vi "Load Dark Array Data.vi"(8 "error in (no error)":errorcluster, 11 "Dark Array Path":path) -> (0 "error out":errorcluster, 1 "Freq":dbl[](array[numeric]), 2 "intTime":dbl[](array[numeric]), 3 "Scans":dbl[][](array[numeric]))   [LabVIEW 2014, in "AvaSpec.lvlib" / "Dark.lvlib"]
uses:
  Dark.lvlib
  AvaSpec.lvlib
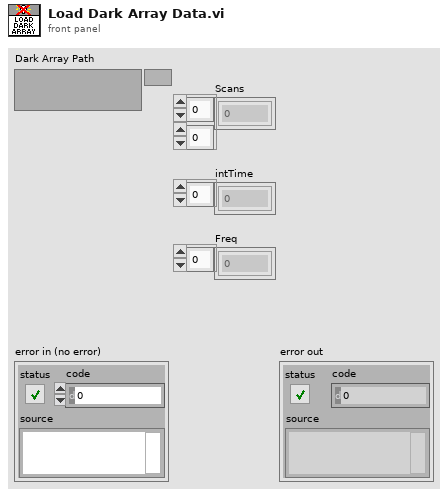
[diagram p1: front panel]
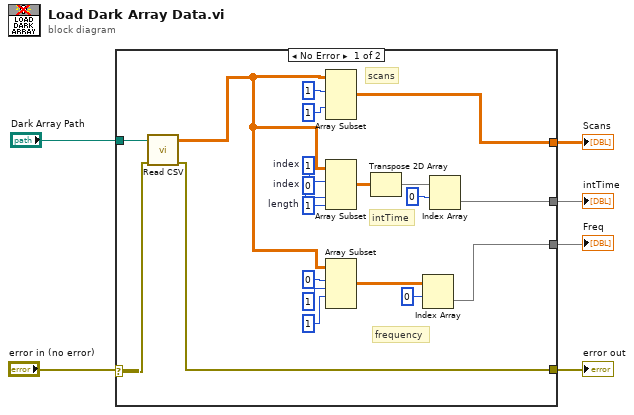
[diagram p0: block diagram]
diagram:
  n1 = case shown="No Error" "error in (no error)" {
    selector: "error in (no error)" -> [w8 w27]
    tunnel: [w26 _] -> w6
    tunnel: [w25 _] -> w5
    tunnel: [w19 _] -> w4
    tunnel: "Dark Array Path" -> [w9 _]
    tunnel: [w7 w27] -> w1
    frame No Error {
      w12 = 0  # index
      w14 = 1  # length
      w11 = 1  # index
      # "scans"
      # "frequency"
      # "intTime"
      n2 = call "Read CSV.vi"("error in (no error)"=w8, "Path"=w9) -> ("error out"=w7:errorcluster, "all rows"=w10:dbl[][])  [unwired: 7 in, 1 out]
      n3 = Array Subset(array=w10, index (row)=1 ("length"), index (col)=1 ("length")) -> (w19:dbl[][])  [unwired: 2 in]
      n4 = Array Subset(array=w10, index (row)=w11, index (col)=w12, length (col)=w14) -> (w23:dbl[][])  [unwired: 1 in]
      n5 = Array Subset(array=w10, index (row)=0 ("length"), length (row)=1 ("length"), index (col)=1 ("length")) -> (w22:dbl[][])  [unwired: 1 in]
      n6 = Transpose 2D Array(2D array=w23) -> (transposed array=w24:dbl[][])
      n7 = Index Array(array=w22, index (row)=0) -> (element=w25:dbl[])  [unwired: 1 in]
      n8 = Index Array(array=w24, index (row)=0) -> (element=w26:dbl[])  [unwired: 1 in]
    }
    frame Error {
    }
  }
  "intTime" <- w6
  "Freq" <- w5
  "Scans" <- w4
  "error out" <- w1
